vi "Get Transceivers.vi"(11 "Framework in":refnum<class "Framework.lvclass">) -> (2 "Transceivers":refnum<class "Transceiver.lvclass">[](array[class]), 3 "Framework out":refnum<class "Framework.lvclass">)   [LabVIEW 2017, in "Data Sharing Framework Core.lvlib" / "Data Sharing Framework Engine.lvlib" / "Framework.lvclass"]
uses:
  Framework.lvclass
  Internal/Transceiver/Transceiver/Transceiver.lvclass
  Framework.lvclass/Framework.ctl
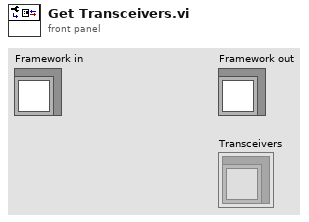
[diagram p1: front panel]
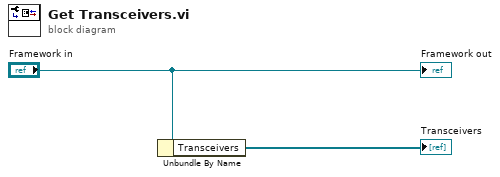
[diagram p0: block diagram]
diagram:
  n1 = Unbundle By Name("Framework in") -> ("Transceivers"=→"Transceivers":refnum<class "Transceiver.lvclass">[])
  "Framework out" <- "Framework in"
